vi "Untitled 2.vi"(9 "RelayCMD":string="Zc", 10 "RelayCtrl":refnum<visa-resource-name>="COM3", 11 "RS485 RECEIVER":refnum<visa-resource-name>="COM1") -> (3 "RECEIVED DATA":string)   [LabVIEW 2011]
uses:
  <vilib>/Instr/_visa.llb/VISA Configure Serial Port (Instr).vi
panel:
  # "F8F0 3EF8 FEFE FE00"
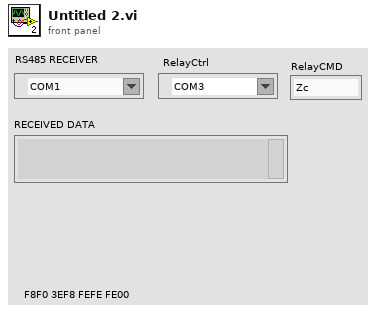
[diagram p1: front panel]
types:
  T1 = enum32{"Set Relay", "Append Relay", "Clear Relay", "Manual Cmd"}
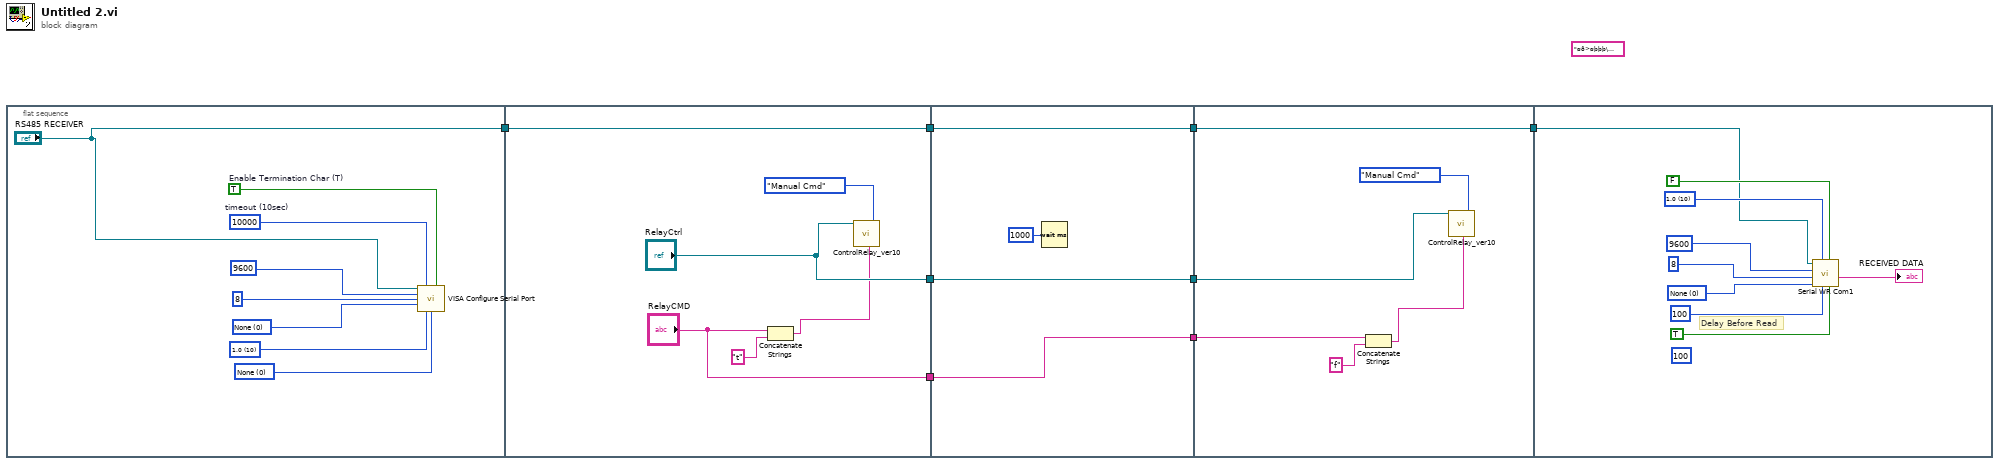
[diagram p0: block diagram]
diagram:
  (unwired) "øð>øþþþ\u0000" ("RECEIVED DATA")
  n1 = flat-sequence {
    tunnel: ["RS485 RECEIVER"] -> w8
    tunnel: [w22] -> w7
    tunnel: w8 -> [w22]
    tunnel: ["RelayCtrl"] -> w3
    tunnel: ["RelayCMD"] -> w1
    tunnel: w7 -> [w26]
    tunnel: [w26] -> w6
    tunnel: [w24] -> w4
    tunnel: w3 -> [w24]
    tunnel: [w23] -> w2
    tunnel: w1 -> [w23]
    tunnel: w6 -> [w32]
    tunnel: [w32] -> w5
    tunnel: w4 -> [w30]
    tunnel: w2 -> [w27]
    tunnel: w5 -> [w34]
    frame #0 {
      w15 = u16 0 items=["None"=0, "XON/XOFF"=1, "RTS/CTS"=2, "DTR/DSR"=4] ("flow control")
      w14 = u16 10 items=["1.0"=10, "1.5"=15, "2.0"=20] ("stop bits")
      w11 = u16 0 items=["None", "Odd", "Even", "Mark", "Space"] ("parity")
      w13 = TRUE  # Enable Termination Char (T)
      w12 = u32 10000  # timeout (10sec)
      n2 = call-poly "VISA Configure Serial Port"("VISA resource name"="RS485 RECEIVER", "timeout (10sec)"=w12, "Enable Termination\nChar (T)"=w13, "baud rate (9600)"=u32 9600, "data bits (8)"=u16 8, "parity (0:none)"=w11, "stop bits (10: 1 bit)"=w14, "flow control (0:none)"=w15) -> ()  [unwired: 1 in, 7 out]
    }
    frame #1 {
      n3 = Concatenate Strings("RelayCMD", "t" ("string")) -> (w19:string)
      n4 = call "ControlRelay_ver10.vi"("VISA session"="RelayCtrl", "write buffer"=w19, "Relay Setting"=T1."Manual Cmd") -> ()  [unwired: 10 in, 7 out]
    }
    frame #2 {
      n5 = Wait (ms)(milliseconds to wait=u32 1000) -> ()  [unwired: 1 out]
    }
    frame #3 {
      n6 = Concatenate Strings(w27, "f" ("string")) -> (w28:string)
      n7 = call "ControlRelay_ver10.vi"("VISA session"=w30, "write buffer"=w28, "Relay Setting"=T1."Manual Cmd") -> ()  [unwired: 10 in, 7 out]
    }
    frame #4 {
      (unwired) u32 100 ("delay before read (ms)")
      w40 = u16 0 items=["None", "Odd", "Even", "Mark", "Space"] ("parity")
      w38 = u16 10 items=["1.0"=10, "1.5"=15, "2.0"=20] ("stop bits")
      # "Delay Before Read"
      n8 = call "Serial WR Com1.vi"("read"=TRUE, "write"=FALSE, "delay before read (ms)"=u32 100, "stop bits"=w38, "parity"=w40, "data bits"=u16 8, "baud rate"=u32 9600, "VISA resource name"=w34) -> ("read string"=→"RECEIVED DATA":string)  [unwired: 2 in, 1 out]
    }
  }
